vi "array view.vi"(8 "i":errorcluster, 11 "array in":refnum<class "Value.lvclass">[](array[class])) -> (0 "o":errorcluster, 3 "array view":T1[](array[typedef]))   [LabVIEW 2023, in "LabGRAD.lvlib" / "Value.lvclass"]
uses:
  Value.lvclass
  value view.ctl
  UiObjects/numeric value control.ctl
  UiObjects/string control.ctl
  operation.ctl
  UiObjects/UiObjects.lvclass
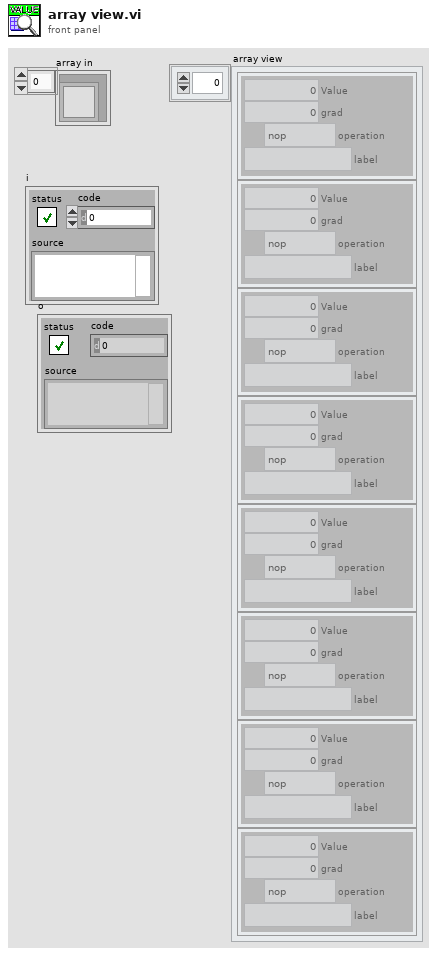
[diagram p1: front panel]
types:
  T1 = typedef "LabGRAD.lvlib/Value.lvclass/value view.ctl" = cluster{"Value":T2, "grad":T2, "label":T3, "operation":T4}
  T2 = typedef "UiObjects.lvlib/UiObjects.lvclass/numeric value control.ctl" = dbl
  T3 = typedef "UiObjects.lvlib/UiObjects.lvclass/string control.ctl" = string
  T4 = typedef "LabGRAD.lvlib/Value.lvclass/operation.ctl" = enum16{"nop", "add", "subtract", "power", "multiply", "divide", "tanh"}
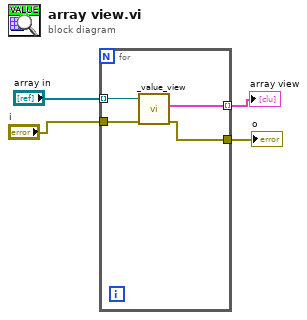
[diagram p0: block diagram]
diagram:
  n1 = for {
    tunnel: "array in" -> [w8] mode=indexing
    tunnel: "i" -> [w7]
    tunnel: [w6] -> w2 mode=indexing
    tunnel: [w5] -> w1
    n2 = call "_value_view.vi"("error in (no error)"=w7, "Value in"=w8) -> ("error out"=w5:errorcluster, "Val View"=w6:T1)  [unwired: 7 in, 1 out]
  }
  "array view" <- w2
  "o" <- w1
